vi "Get 1D Fourier Coefficients.vi"(9 "Period":i32, 10 "Signal":dbl[](array[numeric]), 11 "#Coefficients":i32) -> (3 "Coefficients":cluster{"A0":dbl, "Am":dbl[], "Bm":dbl[]})   [LabVIEW 2020]
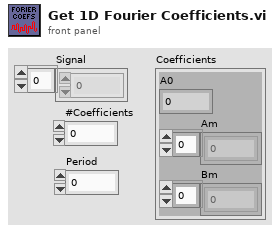
[diagram p1: front panel]
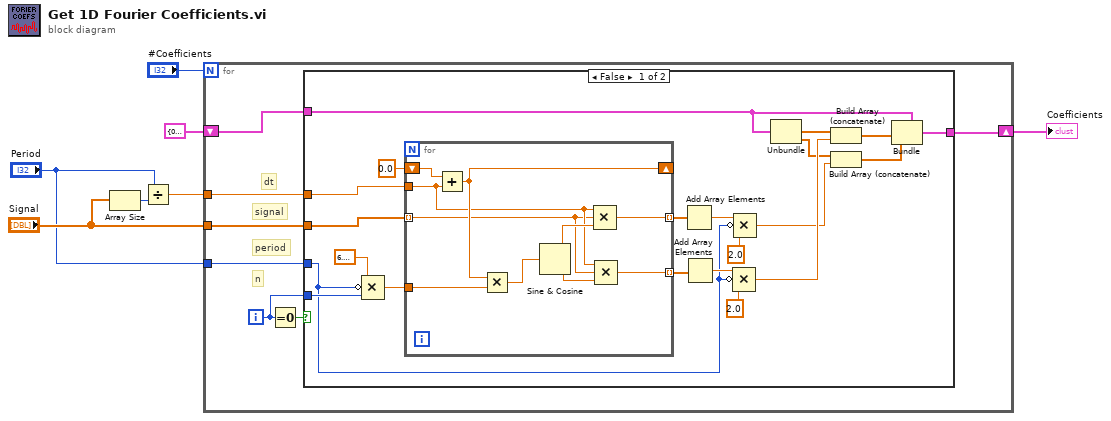
[diagram p0: block diagram]
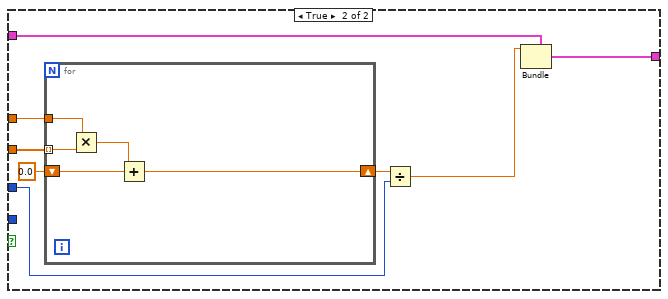
[diagram p2: hidden frame]
diagram:
  n1 = Array Size(array="Signal") -> (size(s)=w4:i32)
  n2 = Divide(x="Period", y=w4) -> (x/y=w1:dbl)
  n3 = for {
    N: "#Coefficients" -> [_]
    tunnel: "Period" -> [w12]
    tunnel: "Signal" -> [w11]
    tunnel: w1 -> [w10]
    shift-right: [w8] -> w7
    shift-left: cluster{"A0":dbl, "Am":dbl[], "Bm":dbl[]} {"A0"=0.0, "Am"=[], "Bm"=[]} ("Cluster") -> [w9]
    i -> [w13]
    # "n"
    # "period"
    # "signal"
    # "dt"
    n4 = Equal To 0?(x=w13) -> (x = 0?=w14:bool)
    n5 = case shown="False" w14 {
      tunnel: w13 -> [w35 _]
      tunnel: w12 -> [w23 w49]
      tunnel: w11 -> [w31 w53]
      tunnel: w10 -> [w32 w51]
      tunnel: w9 -> [w18 w48]
      tunnel: [w15 w46] -> w8
      frame False {
        n6 = Compound Arithmetic op=MULTIPLY(6.283185307179586, invert w23, w35) -> (w33:dbl)
        n7 = for {
          tunnel: w33 -> [w44]
          shift-right: [w43] -> _
          shift-left: 0.0 -> [w45]
          tunnel: w32 -> [w39]
          tunnel: w31 -> [w38] mode=indexing
          tunnel: [w40] -> w29 mode=indexing
          tunnel: [w36] -> w26 mode=indexing
          n8 = Add(x=w45, y=w39) -> (x+y=w43:dbl)
          n9 = Multiply(x=w43, y=w44) -> (x*y=w42:dbl)
          n10 = Sine & Cosine(0:w42) -> (1:w41:dbl, 2:w37:dbl)
          n11 = Compound Arithmetic op=MULTIPLY(w39, w38, w41) -> (w40:dbl)
          n12 = Compound Arithmetic op=MULTIPLY(w39, w38, w37) -> (w36:dbl)
        }
        n13 = Add Array Elements(numeric array=w29) -> (sum=w28:dbl)
        n14 = Add Array Elements(numeric array=w26) -> (sum=w24:dbl)
        n15 = Compound Arithmetic op=MULTIPLY(w24, invert w23, 2.0 ("value")) -> (w21:dbl)
        n16 = Compound Arithmetic op=MULTIPLY(w28, invert w23, 2.0 ("value")) -> (w19:dbl)
        n17 = Unbundle(w18) -> ("Am"=w22:dbl[], "Bm"=w20:dbl[])  [unwired: 1 out]
        n18 = Build Array (concatenate)(w22, w21) -> (w17:dbl[])
        n19 = Build Array (concatenate)(w20, w19) -> (w16:dbl[])
        n20 = Bundle(cluster=w18, "Am"=w17, "Bm"=w16) -> (w15:cluster{"A0":dbl, "Am":dbl[], "Bm":dbl[]})  [unwired: 1 in]
      }
      frame True {
        n21 = for {
          tunnel: w53 -> [w57] mode=indexing
          shift-right: [w58] -> w50
          shift-left: 0.0 -> [w55]
          tunnel: w51 -> [w56]
          n22 = Multiply(x=w56, y=w57) -> (x*y=w54:dbl)
          n23 = Add(x=w54, y=w55) -> (x+y=w58:dbl)
        }
        n24 = Divide(x=w50, y=w49) -> (x/y=w47:dbl)
        n25 = Bundle(cluster=w48, "A0"=w47) -> (w46:cluster{"A0":dbl, "Am":dbl[], "Bm":dbl[]})  [unwired: 2 in]
      }
    }
  }
  "Coefficients" <- w7
